vi "split_num_uint32_t_1.vi"(10 "read_frame":string, 11 "id (2 characters)":string) -> (3 "num_uint32_t":u32)   [LabVIEW 2020]
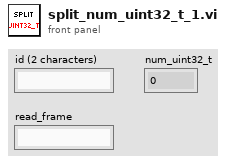
[diagram p1: front panel]
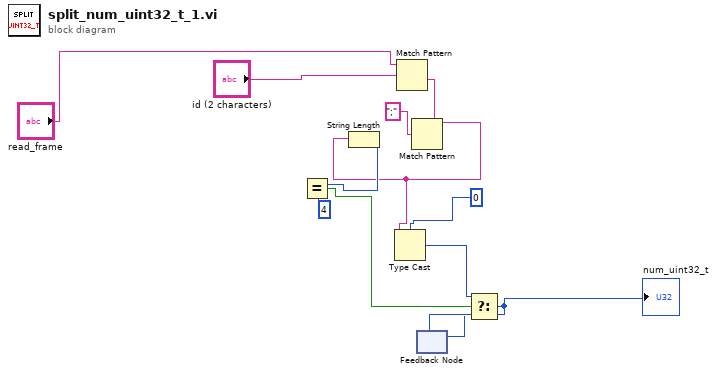
[diagram p0: block diagram]
diagram:
  n1 = Match Pattern(string="read_frame", regular expression="id (2 characters)") -> (after substring=w1:string)  [unwired: 1 in, 3 out]
  n2 = Match Pattern(string=w1, regular expression=";") -> (before substring=w7:string)  [unwired: 1 in, 3 out]
  n3 = String Length(string=w7) -> (length=w8:i32)
  n4 = Equal?(x=w8, y=4) -> (x = y?=w10:bool)
  n5 = Type Cast(type=u32 0, x=w7) -> (*(type *) &x=w4:u32)
  n6 = feedback #1() -> (w5:u32)  [unwired: 1 in]
  n7 = Select(t=w4, s=w10, f=w5) -> (s? t:f=w11:u32)
  "num_uint32_t" <- w11
  n8 = feedback-in #1(w11) -> ()
